vi "Send command Set Port.vi"(7 "Marca":string, 8 "error in (no error)":errorcluster, 9 "Valor HEX":string, 10 "Puerto":string, 11 "NXP in":refnum<class "NXP.lvclass">) -> (0 "error out":errorcluster, 1 "Command":string, 2 "Expected response":string, 3 "NXP out":refnum<class "NXP.lvclass">)   [LabVIEW 2020, in "NXP.lvclass"]
uses:
  NXP.lvclass
  NXP.lvclass/NXP.ctl
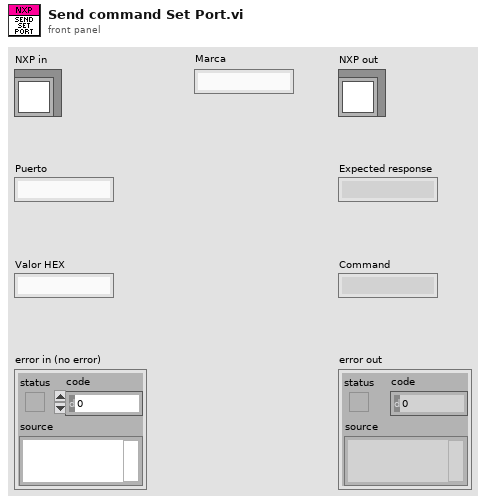
[diagram p1: front panel]
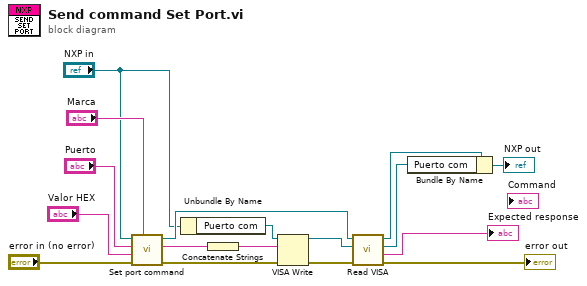
[diagram p0: block diagram]
diagram:
  n1 = call-dynamic "Set port command.vi"("Marca"="Marca", "error in (no error)"="error in (no error)", "Valor HEX"="Valor HEX", "Puerto"="Puerto", "Serial Device in"="NXP in") -> ("error out"=w12:errorcluster, "Command"=w8:string, "Serial Device out"=w10:refnum<class "NXP.lvclass">)  [unwired: 3 in, 1 out]
  n2 = Unbundle By Name("NXP in") -> ("Puerto com"=w6:refnum<visa-resource-name>)
  n3 = Concatenate Strings(w8) -> (w9:string)
  n4 = VISA Write(VISA resource name=w6, write buffer=w9, error in (no error)=w12) -> (VISA resource name out=w5:refnum<visa-resource-name>, error out=w13:errorcluster)  [unwired: 1 out]
  n5 = call-dynamic "Read VISA.vi"("error in (no error)"=w13, "VISA Refnum in"=w5, "Serial Device in"=w10) -> ("error out"=→"error out":errorcluster, "Serial Response"=→"Expected response":string, "VISA resource name out"=w2:refnum<visa-resource-name>, "Serial Device out"=w4:refnum<class "NXP.lvclass">)  [unwired: 5 in]
  n6 = Bundle By Name(cluster=w4, "Puerto com"=w2) -> (→"NXP out":refnum<class "NXP.lvclass">)
